vi "findVisaResources.vi"(8 "error in (no error)":errorcluster) -> (0 "error out":errorcluster, 3 "find list":string[](array[string]))   [LabVIEW 2018]
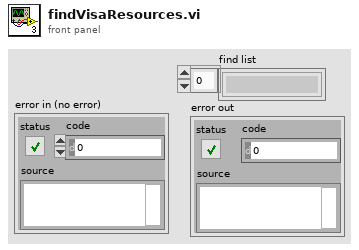
[diagram p1: front panel]
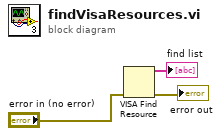
[diagram p0: block diagram]
diagram:
  n1 = VISA Find Resource(8:"error in (no error)") -> (0:→"error out":errorcluster, 3:→"find list":string[])  [unwired: 2 in, 1 out]
